vi "Update-acquisition-status.vi"(7 "Tigger ok?":bool, 8 "error in (no error)":errorcluster, 9 "Queue ok?":bool, 10 "Image ok?":bool, 11 "Acquis. params. ref. in":refnum<data-value>) -> (0 "error out":errorcluster, 3 "Acquis. params. ref.":refnum<data-value>)   [LabVIEW 2013, in "CameraVision.lvlib" / "CV-Acquisition.lvclass"]
uses:
  CV-Acquisition.lvclass
  CV-Acquisition.lvclass/CV-Acquisition.ctl
  UI/Module-states.ctl
  Write Acquisition status.vi
  Read Acquisition status.vi
  UI/CV-UI.lvclass
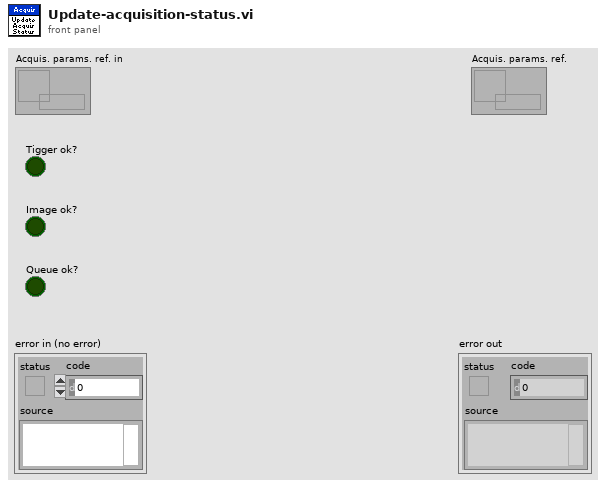
[diagram p1: front panel]
types:
  T1 = typedef "Module-status.ctl" = enum16{"Inactive", "Active", "Data-loss", "Error", "Simulation", "Synchronizing", "Initialized", "Released"}
  T2 = typedef "CameraVision.lvlib/CV-UI.lvclass/Module-states.ctl" = enum16{"Inactive", "Active", "Data-loss", "Error", "Simulation", "Synchronizing", "Initialized", "Released"}
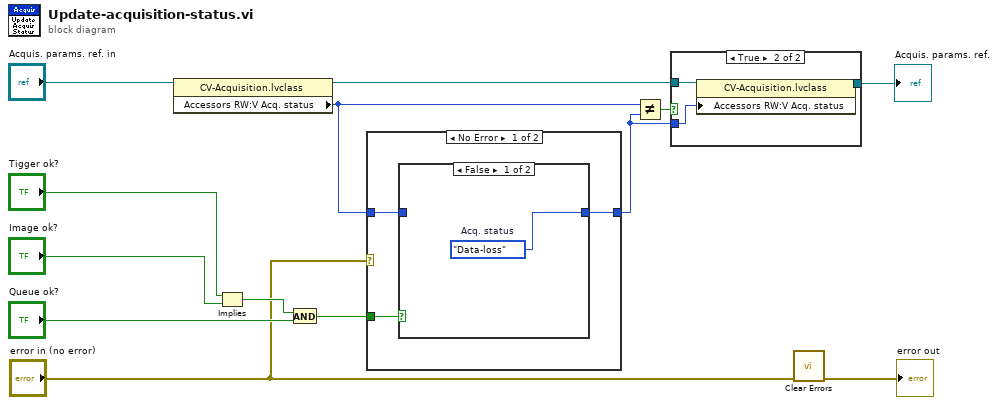
[diagram p0: block diagram]
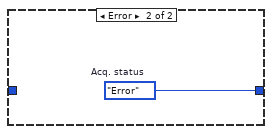
[diagram p4: hidden frame]
diagram:
  n1 = property class="CV-Acquisition.lvclass"(reference="Acquis. params. ref. in") -> (reference out=w10:refnum<data-value>, "Accessors RW:V Acq. status"=w3:T1)  [unwired: 1 in, 1 out]
  n2 = Implies(1:"Image ok?", 2:"Tigger ok?") -> (0:w5:bool)
  n3 = And(x=w5, y="Queue ok?") -> (x .and. y?=w6:bool)
  n4 = case shown="No Error" "error in (no error)" {
    tunnel: w3 -> [w15 _]
    tunnel: w6 -> [w16 _]
    tunnel: [w14 w19] -> w2
    frame No Error {
      n5 = case shown="False" w16 {
        tunnel: w15 -> [_ w18]
        tunnel: [w17 w18] -> w14
        frame False {
          w17 = Module-states."Data-loss"  # Acq. status
        }
        frame True {
        }
      }
    }
    frame Error {
      w19 = Module-states."Error"  # Acq. status
    }
  }
  n6 = Not Equal?(x=w3, y=w2) -> (x != y?=w4:bool)
  n7 = case shown="True" w4 {
    tunnel: [w20 w23] -> w11
    tunnel: w10 -> [w20 w22]
    tunnel: w2 -> [_ w21]
    frame False {
    }
    frame True {
      n8 = property class="CV-Acquisition.lvclass"(reference=w22, "Accessors RW:V Acq. status"=w21) -> (reference out=w23:refnum<data-value>)  [unwired: 1 in, 1 out]
    }
  }
  "Acquis. params. ref." <- w11
  n9 = call <vilib>:"Clear Errors.vi"("error in (no error)"="error in (no error)") -> ("error out"=→"error out":errorcluster)  [unwired: 6 in]
